vi "BLFind_ConvertData.vi"(10 "pNbrDev":u32, 11 "pLstdev":u8[](array[numeric])) -> (3 "device table":string[][](table))   [LabVIEW 2022 SP3, in "EClib functions.lvlib"]
uses:
  EClib functions.lvlib
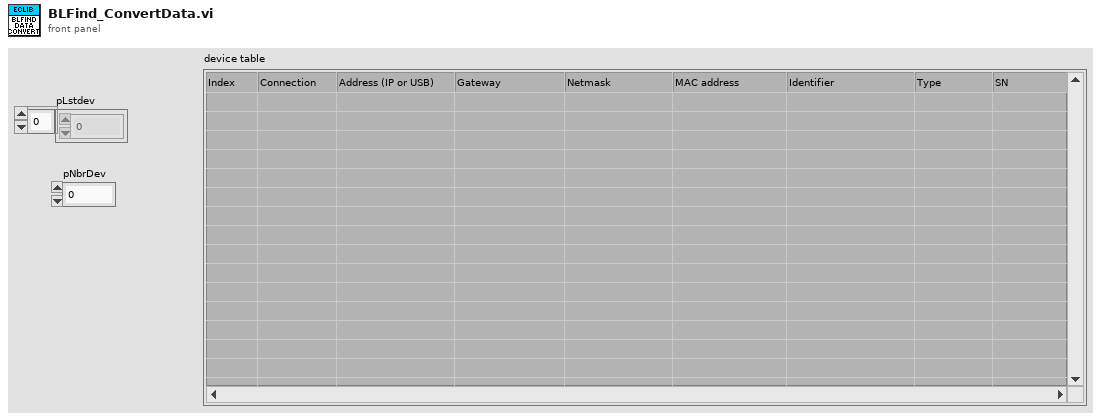
[diagram p1: front panel]
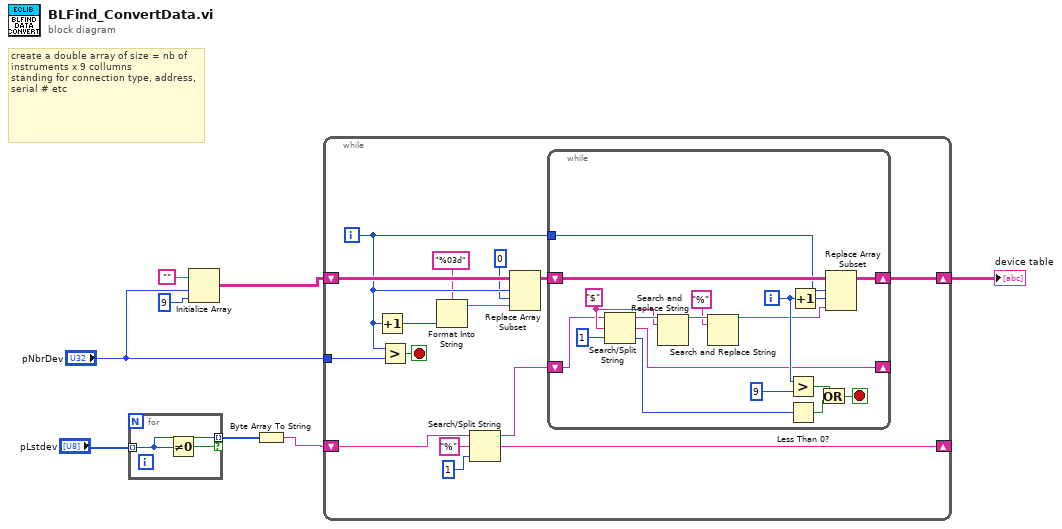
[diagram p0: block diagram]
diagram:
  # "create a double array of size = nb of instruments x 9 collumns \nstanding for connection type, address, serial # etc"
  n1 = for {
    tunnel: "pLstdev" -> [w9] mode=indexing
    tunnel: [w9] -> w3 mode=indexing if=w10
    n2 = Not Equal To 0?(x=w9) -> (x != 0?=w10:bool)
  }
  n3 = Initialize Array("", "pNbrDev", 9 ("dimension size")) -> (w5:string[][])
  n4 = Byte Array To String(unsigned byte array=w3) -> (string=w1:string)
  n5 = while {
    tunnel: "pNbrDev" -> [w18]
    shift-right: [w21] -> _
    shift-left: w1 -> [w22]
    shift-right: [w20] -> w4
    shift-left: w5 -> [w17]
    i -> [w15]
    stop <- w25 stop-if-true
    n6 = Increment(x=w15) -> (x+1=w12:i32)
    n7 = Greater?(x=w15, y=w18) -> (0:w25:bool)
    n8 = Format Into String(format string="%03d", w12) -> (resulting string=w13:string)  [unwired: 2 in, 1 out]
    n9 = Search/Split String(string=w22, search string/char (-)="%", offset (0)=1) -> (substring before match=w23:string, match + rest of string=w21:string)  [unwired: 1 out]
    n10 = Replace Array Subset(array=w17, new element=w13, index (row)=w15, index (col)=0 ("disabled index (col)")) -> (w16:string[][])
    n11 = while {
      tunnel: w15 -> [w31]
      shift-right: [w28] -> _
      shift-left: w23 -> [w27]
      shift-right: [w38] -> w20
      shift-left: w16 -> [w42]
      i -> [w37]
      stop <- w39 stop-if-true
      w29 = "$"
      n12 = Search/Split String(string=w27, search string/char (-)=w29, offset (0)=1) -> (substring before match=w34:string, match + rest of string=w28:string, offset of match=w43:i32)
      n13 = Search and Replace String(input string=w34, search string=w29) -> (result string=w33:string)  [unwired: 6 in, 3 out]
      n14 = Search and Replace String(input string=w33, search string="%") -> (result string=w26:string)  [unwired: 6 in, 3 out]
      n15 = Greater?(x=w37, y=9) -> (0:w41:bool)
      n16 = Less Than 0?(x=w43) -> (x < 0?=w40:bool)
      n17 = Increment(x=w37) -> (x+1=w30:i32)
      n18 = Or(x=w41, y=w40) -> (x .or. y?=w39:bool)
      n19 = Replace Array Subset(array=w42, new element=w26, index (row)=w31, index (col)=w30) -> (w38:string[][])
    }
  }
  "device table" <- w4
